vi "tic_tac_toe.vi"() -> ()   [LabVIEW 2020]
uses:
  ENUM.ctl
panel:
  in  "RESET":bool
  out "PLAYER":string
  out "Array 2":string[][](array[string])
  in  "Person Slide Switch":bool
  in  "Array":bool[][](array[boolean])
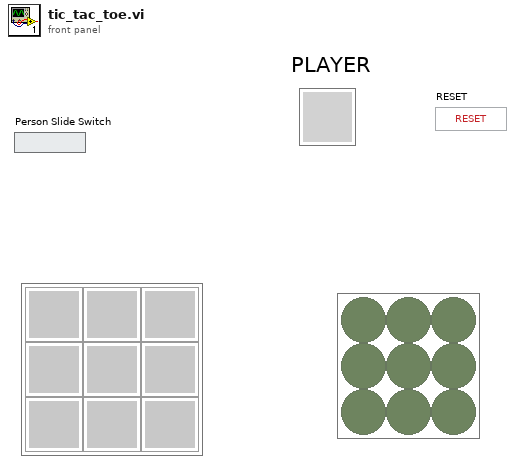
[diagram p1: front panel]
types:
  T1 = typedef "ENUM.ctl" = enum16{"INIT", "START", "WINNER_STATUS", "WINNER", "STOP", "RESET"}
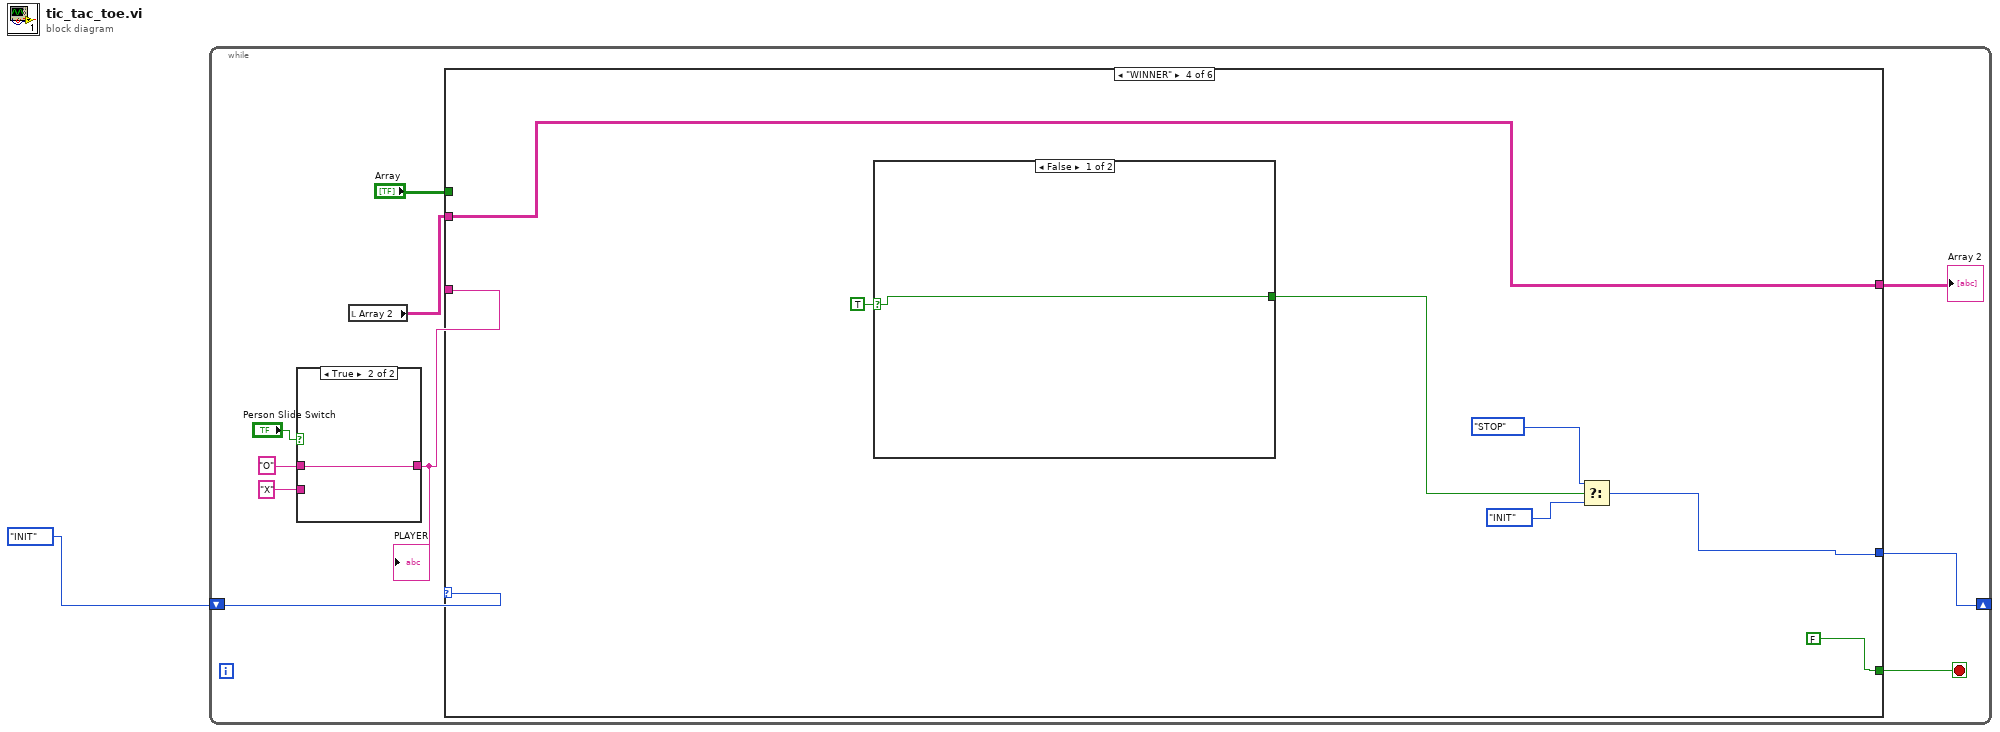
[diagram p0: block diagram]
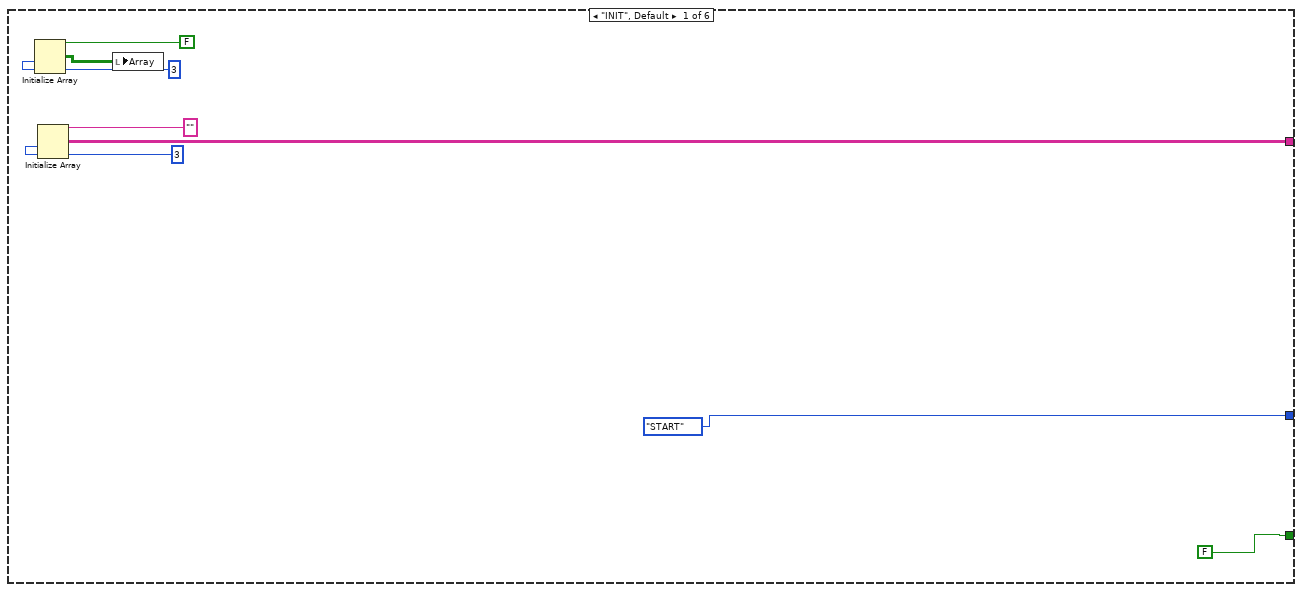
[diagram p3: hidden frame]
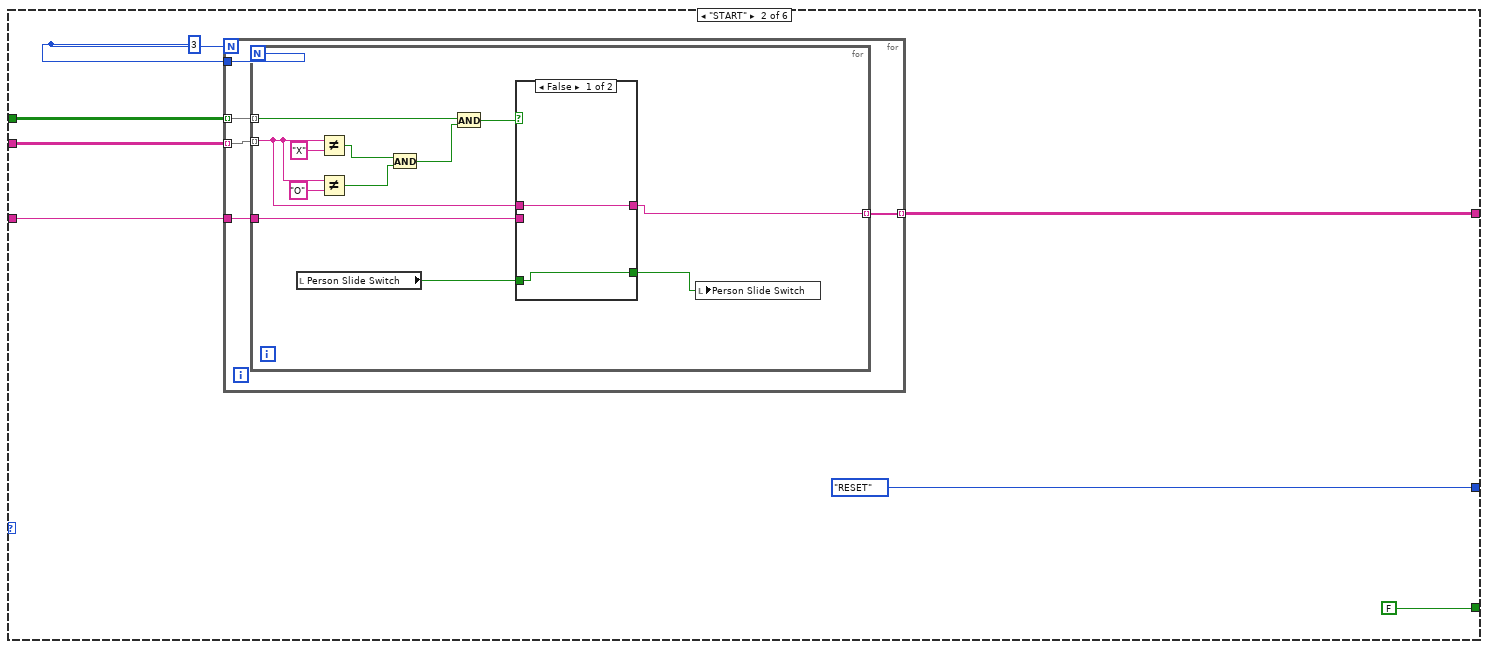
[diagram p4: hidden frame]
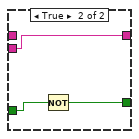
[diagram p5: hidden frame]
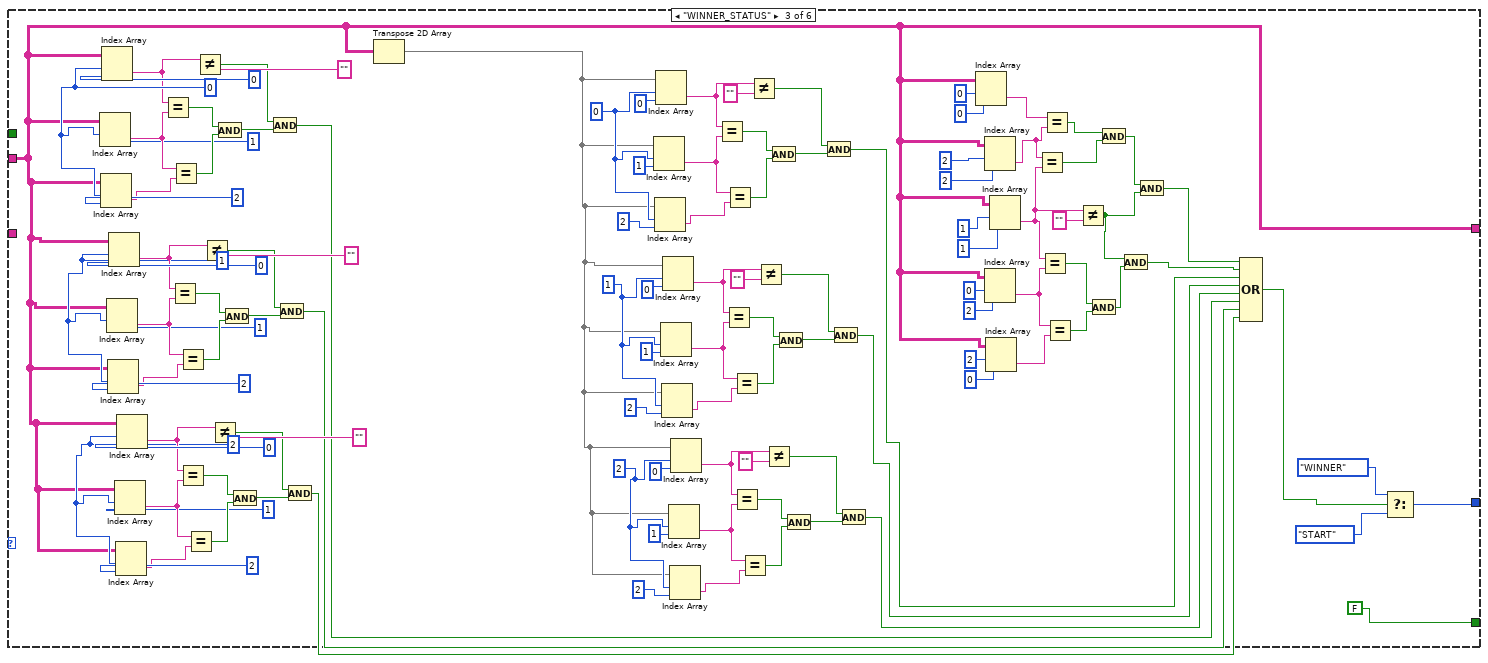
[diagram p6: hidden frame]
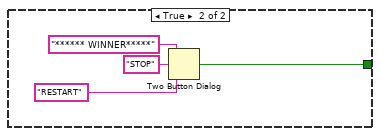
[diagram p7: hidden frame]
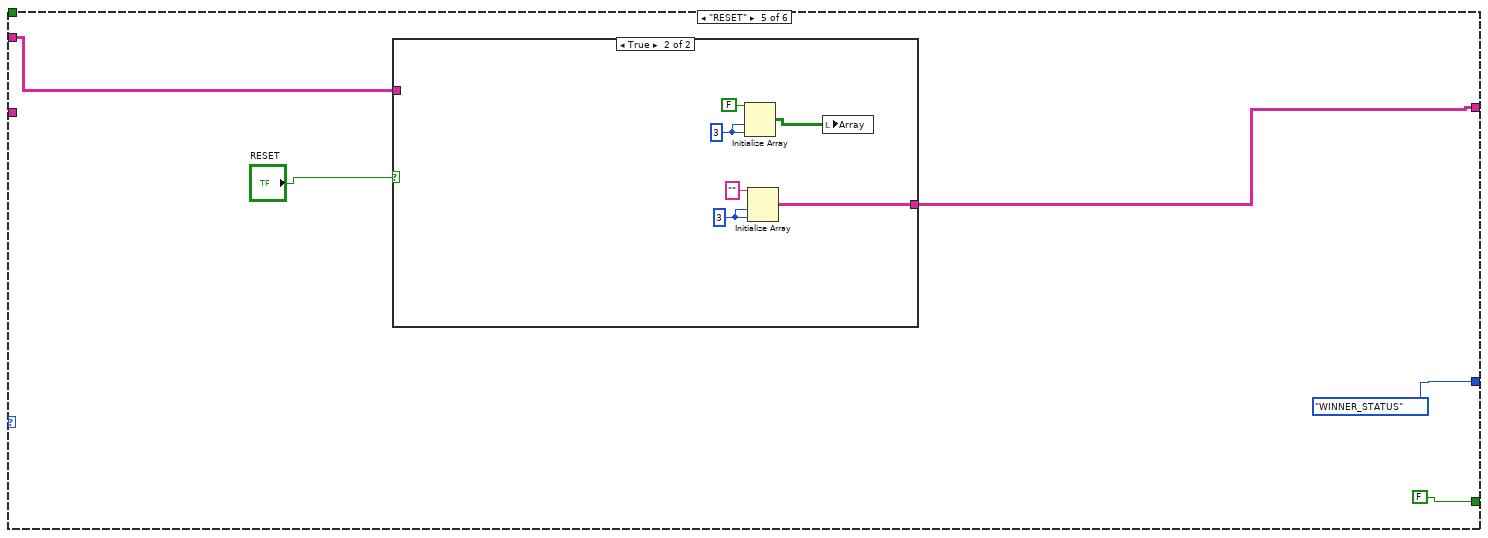
[diagram p8: hidden frame]
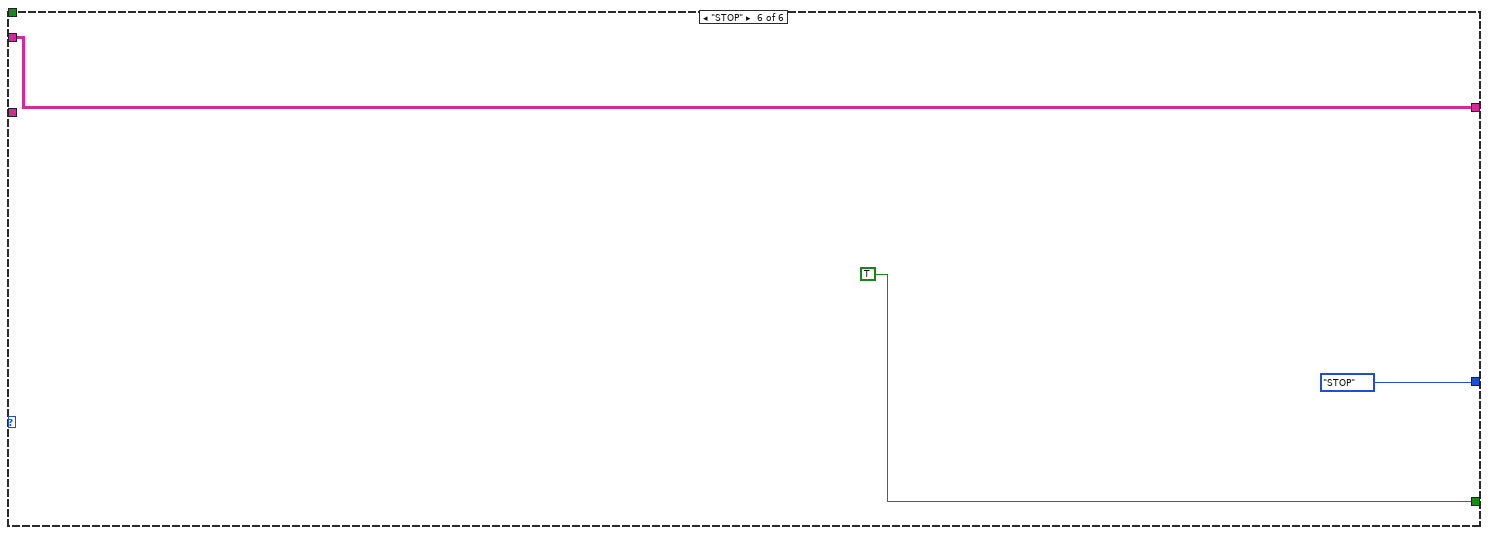
[diagram p10: hidden frame]
diagram:
  n1 = while {
    shift-right: [w5] -> _
    shift-left: ENUM."INIT" -> [w11]
    stop <- w2 stop-if-true
    n2 = case shown="True" "Person Slide Switch" {
      tunnel: "O" -> [_ w13]
      tunnel: "X" -> [w12 _]
      tunnel: [w12 w13] -> w7
      frame False {
      }
      frame True {
      }
    }
    "PLAYER" <- w7
    n3 = local read "Array 2"() -> (w4:string[][])
    n4 = case shown="\"WINNER\"" w11 {
      tunnel: w7 -> [_ w24 _ _ _ _]
      tunnel: [w16 w25 w83 w161 w176 w185] -> w3
      tunnel: "Array" -> [_ w27 _ _ _ _]
      tunnel: w4 -> [_ w26 w83 w161 w175 w185]
      tunnel: [ENUM."START" ENUM."RESET" w59 w163 ENUM."WINNER_STATUS" ENUM."STOP"] -> w5
      tunnel: [FALSE FALSE FALSE FALSE FALSE TRUE] -> w2
      frame "INIT", Default {
        w17 = 3 ("dimension size")
        w19 = 3 ("dimension size")
        n5 = Initialize Array(FALSE, w19, w19) -> (w20:bool[][])
        n6 = Initialize Array("", w17, w17) -> (w16:string[][])
        n7 = local write "Array"(w20) -> ()
      }
      frame "START" {
        w28 = 3
        n8 = for {
          N: w28 -> [_]
          tunnel: w28 -> [w33]
          tunnel: w27 -> [w32] mode=indexing
          tunnel: w26 -> [w31] mode=indexing
          tunnel: [w30] -> w25 mode=indexing
          tunnel: w24 -> [w29]
          n9 = for {
            N: w33 -> [_]
            tunnel: w32 -> [w43] mode=indexing
            tunnel: w31 -> [w36] mode=indexing
            tunnel: [w35] -> w30 mode=indexing
            tunnel: w29 -> [w34]
            n10 = local read "Person Slide Switch"() -> (w45:bool)
            n11 = Not Equal?(x=w36, y="X") -> (x != y?=w40:bool)
            n12 = Not Equal?(x=w36, y="O") -> (x != y?=w39:bool)
            n13 = And(x=w40, y=w39) -> (x .and. y?=w38:bool)
            n14 = And(x=w43, y=w38) -> (x .and. y?=w37:bool)
            n15 = case shown="False" w37 {
              tunnel: w45 -> [w46 w50]
              tunnel: [w46 w49] -> w44
              tunnel: [w47 w48] -> w35
              tunnel: w36 -> [w47 _]
              tunnel: w34 -> [_ w48]
              frame False {
              }
              frame True {
                n16 = Not(x=w50) -> (.not. x?=w49:bool)
              }
            }
            n17 = local write "Person Slide Switch"(w44) -> ()
          }
        }
      }
      frame "WINNER_STATUS" {
        w95 = 2
        w106 = 1
        w126 = 0 ("index (row)")
        w128 = 2
        w139 = 1
        w159 = 0 ("index (row)")
        n18 = Index Array(array=w83, index (row)=w159, index (col)=1 ("disabled index (col)")) -> (element=w157:string)
        n19 = Index Array(array=w83, index (row)=w159, index (col)=2 ("disabled index (col)")) -> (element=w156:string)
        n20 = Index Array(array=w83, index (row)=w159, index (col)=0 ("disabled index (col)")) -> (element=w155:string)
        n21 = Index Array(array=w83, index (row)=w139, index (col)=1 ("disabled index (col)")) -> (element=w147:string)
        n22 = Index Array(array=w83, index (row)=w139, index (col)=2 ("disabled index (col)")) -> (element=w146:string)
        n23 = Index Array(array=w83, index (row)=w139, index (col)=0 ("disabled index (col)")) -> (element=w145:string)
        n24 = Index Array(array=w83, index (row)=w128, index (col)=1 ("disabled index (col)")) -> (element=w136:string)
        n25 = Index Array(array=w83, index (row)=w128, index (col)=2 ("disabled index (col)")) -> (element=w135:string)
        n26 = Index Array(array=w83, index (row)=w128, index (col)=0 ("disabled index (col)")) -> (element=w134:string)
        n27 = Equal?(x=w155, y=w157) -> (x = y?=w153:bool)
        n28 = Equal?(x=w145, y=w147) -> (x = y?=w143:bool)
        n29 = Equal?(x=w157, y=w156) -> (x = y?=w152:bool)
        n30 = Equal?(x=w147, y=w146) -> (x = y?=w142:bool)
        n31 = Equal?(x=w134, y=w136) -> (x = y?=w132:bool)
        n32 = Equal?(x=w136, y=w135) -> (x = y?=w131:bool)
        n33 = Not Equal?(x=w155, y="") -> (x != y?=w150:bool)
        n34 = Not Equal?(x=w145, y="") -> (x != y?=w140:bool)
        n35 = Not Equal?(x=w134, y="") -> (x != y?=w129:bool)
        n36 = And(x=w153, y=w152) -> (x .and. y?=w151:bool)
        n37 = And(x=w143, y=w142) -> (x .and. y?=w141:bool)
        n38 = And(x=w132, y=w131) -> (x .and. y?=w130:bool)
        n39 = And(x=w150, y=w151) -> (x .and. y?=w67:bool)
        n40 = And(x=w140, y=w141) -> (x .and. y?=w68:bool)
        n41 = And(x=w129, y=w130) -> (x .and. y?=w69:bool)
        n42 = Transpose 2D Array(2D array=w83) -> (transposed array=w94:string[][])
        n43 = Index Array(array=w94, index (row)=w126, index (col)=1 ("disabled index (col)")) -> (element=w124:string)
        n44 = Index Array(array=w94, index (row)=w126, index (col)=2 ("disabled index (col)")) -> (element=w123:string)
        n45 = Index Array(array=w94, index (row)=w126, index (col)=0 ("disabled index (col)")) -> (element=w122:string)
        n46 = Index Array(array=w94, index (row)=w106, index (col)=1 ("disabled index (col)")) -> (element=w114:string)
        n47 = Index Array(array=w94, index (row)=w106, index (col)=2 ("disabled index (col)")) -> (element=w113:string)
        n48 = Index Array(array=w94, index (row)=w106, index (col)=0 ("disabled index (col)")) -> (element=w112:string)
        n49 = Index Array(array=w94, index (row)=w95, index (col)=1 ("disabled index (col)")) -> (element=w103:string)
        n50 = Index Array(array=w94, index (row)=w95, index (col)=2 ("disabled index (col)")) -> (element=w102:string)
        n51 = Index Array(array=w94, index (row)=w95, index (col)=0 ("disabled index (col)")) -> (element=w101:string)
        n52 = Equal?(x=w122, y=w124) -> (x = y?=w120:bool)
        n53 = Equal?(x=w112, y=w114) -> (x = y?=w110:bool)
        n54 = Equal?(x=w124, y=w123) -> (x = y?=w119:bool)
        n55 = Equal?(x=w114, y=w113) -> (x = y?=w109:bool)
        n56 = Equal?(x=w101, y=w103) -> (x = y?=w99:bool)
        n57 = Equal?(x=w103, y=w102) -> (x = y?=w98:bool)
        n58 = Not Equal?(x=w122, y="") -> (x != y?=w117:bool)
        n59 = Not Equal?(x=w112, y="") -> (x != y?=w107:bool)
        n60 = Not Equal?(x=w101, y="") -> (x != y?=w96:bool)
        n61 = And(x=w120, y=w119) -> (x .and. y?=w118:bool)
        n62 = And(x=w110, y=w109) -> (x .and. y?=w108:bool)
        n63 = And(x=w99, y=w98) -> (x .and. y?=w97:bool)
        n64 = And(x=w117, y=w118) -> (x .and. y?=w64:bool)
        n65 = And(x=w107, y=w108) -> (x .and. y?=w65:bool)
        n66 = And(x=w96, y=w97) -> (x .and. y?=w66:bool)
        n67 = Index Array(array=w83, index (row)=0, index (col)=0 ("disabled index (col)")) -> (element=w79:string)
        n68 = Index Array(array=w83, index (row)=2, index (col)=2 ("disabled index (col)")) -> (element=w80:string)
        n69 = Index Array(array=w83, index (row)=0, index (col)=2 ("disabled index (col)")) -> (element=w82:string)
        n70 = Index Array(array=w83, index (row)=2, index (col)=0 ("disabled index (col)")) -> (element=w81:string)
        n71 = Index Array(array=w83, index (row)=1, index (col)=1 ("disabled index (col)")) -> (element=w77:string)
        n72 = Equal?(x=w80, y=w77) -> (x = y?=w75:bool)
        n73 = Equal?(x=w77, y=w82) -> (x = y?=w72:bool)
        n74 = Equal?(x=w79, y=w80) -> (x = y?=w76:bool)
        n75 = Equal?(x=w82, y=w81) -> (x = y?=w71:bool)
        n76 = Not Equal?(x=w77, y="") -> (x != y?=w73:bool)
        n77 = And(x=w72, y=w71) -> (x .and. y?=w70:bool)
        n78 = And(x=w76, y=w75) -> (x .and. y?=w74:bool)
        n79 = And(x=w73, y=w70) -> (x .and. y?=w63:bool)
        n80 = And(x=w74, y=w73) -> (x .and. y?=w62:bool)
        n81 = Compound Arithmetic op=OR(w62, w63, w64, w65, w66, w67, w68, w69) -> (w58:bool)
        n82 = Select(t=ENUM."WINNER", s=w58, f=ENUM."START") -> (s? t:f=w59:T1)
      }
      frame "WINNER" {
        n83 = case shown="False" TRUE {
          selector: TRUE -> [w168 _]
          tunnel: [w168 w169] -> w166
          frame False {
          }
          frame True {
            n84 = Two Button Dialog(message="****** WINNER*****", 1:"RESTART" ("F button name (\"Cancel\")"), 2:"STOP" ("T button name (\"OK\")")) -> (T button?=w169:bool)
          }
        }
        n85 = Select(t=ENUM."STOP", s=w166, f=ENUM."INIT") -> (s? t:f=w163:T1)
      }
      frame "RESET" {
        n86 = case shown="True" "RESET" {
          tunnel: [w178 w179] -> w176
          tunnel: w175 -> [w178 _]
          frame False {
          }
          frame True {
            w180 = 3 ("dimension size")
            w182 = 3 ("dimension size")
            n87 = Initialize Array(FALSE, w182, w182) -> (w183:bool[][])
            n88 = Initialize Array("", w180, w180) -> (w179:string[][])
            n89 = local write "Array"(w183) -> ()
          }
        }
      }
      frame "STOP" {
      }
    }
    "Array 2" <- w3
  }
